vi "FTW-CodeGen-UpdateCodegenCache.vi"(5 "FTW XNode State":T1 {"TotalCodeGens" format="CodeGens:   %04d"; "TotalAdaptToInputs" format="AdaptTerms: %04d"; "FinishedCodegen" format="%_3psec"; "ElapsedTilCodegen" format="%_3psec"; "AdaptToInputsBegin" format="%.3fmsec\n%<%D:%H:%M:%S%3u>t"}, 7 "CodeGen Begin Timer":dbl format="%.3fmsec\n%<%D:%H:%M:%S%3u>t", 11 "error in":errorcluster) -> (6 "FTW XNode State out":T1 {"TotalCodeGens" format="CodeGens:   %04d"; "TotalAdaptToInputs" format="AdaptTerms: %04d"; "FinishedCodegen" format="%_3psec"; "ElapsedTilCodegen" format="%_3psec"; "AdaptToInputsBegin" format="%.3fmsec\n%<%D:%H:%M:%S%3u>t"})   [LabVIEW 2015]
uses:
  FTW-CodeGen-XNodeCommonState.ctl
  FTW-CodeGen-XNodeAdaptiveTerminal.ctl
  FTW-CodeGen-XNodeAdaptiveTerminal-Controller.ctl
  src/reflection/FTW-Reflection-Types.ctl
  FTW-CodeGen-XNodeAdaptiveTerminal-ControllerBehavior.ctl
  src/error/FTW-ERR-NoErrorConstant.vi
  lib/FTW-KernelFilepath.vi
panel:
  # "Inputs"
  # "Outputs"
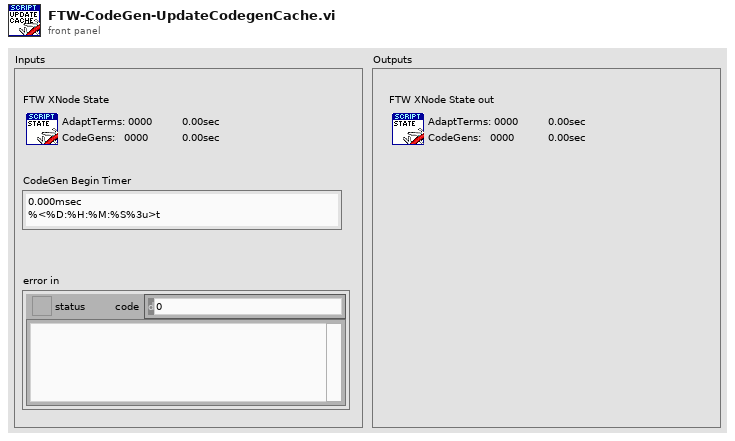
[diagram p1: front panel]
types:
  T1 = typedef "FTW-CodeGen-XNodeCommonState.ctl" = cluster{"Terms":cluster{"Name":string, "Id":string, "Type":variant, "Bounds":cluster{"Left":i32, "Top":i32, "Right":i32, "Bottom":i32}, "Input?":bool, "Required?":bool, "Recommended?":bool, "Adaptive?":bool, "Hidden?":bool, "Direction":enum32{"Auto", "Up", "Down", "Left", "Right", "Center"}, "Break Wire?":bool, "English Name":string}[], "AdaptiveTerms":T2[], "AdaptiveTerminalsOK":bool, "ForceCodeRegeneration?":bool, "LastGeneration":timestamp, "CodeGenError":errorcluster, "AdaptToInputsBegin":dbl, "ElapsedTilCodegen":dbl, "FinishedCodegen":dbl, "TotalAdaptToInputs":i32, "TotalCodeGens":i32}
  T2 = typedef "FTW-CodeGen-XNodeAdaptiveTerminal.ctl" = cluster{"Config":T3, "ID":string, "ParentIndex":i32, "Wired?":bool, "WiredTypeAllowed?":bool, "LastValidWireName":string, "LastValidWireType":T4, "Followers":i32[]}
  T3 = typedef "FTW-CodeGen-XNodeAdaptiveTerminal-Controller.ctl" = cluster{"AllowedTypes":T4[], "UnconstrainedTypeBehavior":T5, "DefaultType":variant}
  T4 = typedef "FTW-Reflection-Types.ctl" = enum16{"Unknown", "Void", "Array", "Cluster", "LVObject", "Boolean", "I8", "I16", "I32", "I64", "U8", "U16", "U32", "U64", "SGL", "DBL", "EXT", "CSG", "CDB", "CXT", "FXP", "EnumU8", "EnumU16", "EnumU32", "EnumU64", "SGLwithUnit", "DBLwithUnit", "EXTwithUnit", "CSGwithUnit", "CDBwithUnit", "CXTwithUnit", "String", "Path", "Picture", "Tag", "LVVariant", "Timestamp", "WaveformI8", "WaveformI16", "WaveformI32", "WaveformI64", "WaveformU8", "WaveformU16", "WaveformU32", "WaveformU64", "WaveformSGL", "WaveformDBL", "WaveformEXT", "WaveformCSG", "WaveformCDB", "WaveformCXT", "WaveformDigital", "WaveformUnknownType", "DigitalData", "DynamicData", "ExternalData", "FileByteStream", "TDMStream", "dotNET", "ActiveX", "VIServerReference", "VIReference", "ApplicationInstance", "Menu", "ConnectionDataSocket", "ConnectionVISA", "ConnectionBluetooth", "ConnectionIrDA", "ConnectionTCP", "ConnectionUDP", "ConnectionHTTPClient", "ConnectionFTP", "Occurrence", "Notifier", "Queue", "Rendezvous", "Semaphore", "RTFIFO", "EventPublisher", "EventRegistration", "EventCallback", "DataValueReference", "GenericClass", "GenericClassTag", "GenericClassDeepCopy", "GenericClassFlattened", "GenericClassTagFlattened", "GenericReferenceType", "WindowsRegistry", "OverloadedDatalogRef", "ReferenceUnknownType", "ByteArray", "ConPaneInterface", "FTWObject"}
  T5 = typedef "FTW-CodeGen-XNodeAdaptiveTerminal-ControllerBehavior.ctl" = enum16{"UseDefaultType", "StickyToLastValidType"}
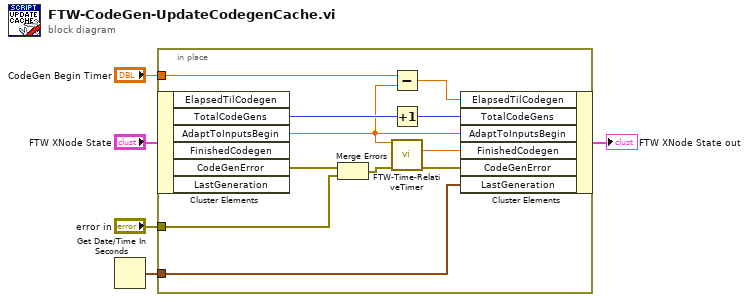
[diagram p0: block diagram]
diagram:
  n1 = Get Date/Time In Seconds() -> (seconds since 1Jan1904=w4:timestamp)
  n2 = in-place {
    in-place-border: w4 -> [w12]
    in-place-border: "error in" -> [w15]
    in-place-border: "CodeGen Begin Timer" -> [w7]
    n3 = in-place-cluster #1("FTW XNode State") -> ("TotalCodeGens"=w10:i32, "AdaptToInputsBegin"=w8:dbl, "CodeGenError"=w16:errorcluster)  [unwired: 3 out]
    n4 = Merge Errors(w16, w15) -> (w14:errorcluster)
    n5 = Subtract(x=w7, y=w8) -> (x-y=w6:dbl)
    n6 = Increment(x=w10) -> (x+1=w9:i32)
    n7 = call "FTW-Time-RelativeTimer.vi"("Previous Timer Value"=w8, "error in"=w14) -> ("Elapsed Time"=w11:dbl, "error out"=w13:errorcluster)  [unwired: 11 in, 1 out]
    n8 = in-place-cluster #1("ElapsedTilCodegen"=w6, "TotalCodeGens"=w9, "AdaptToInputsBegin"=w8, "FinishedCodegen"=w11, "CodeGenError"=w13, "LastGeneration"=w12) -> (→"FTW XNode State out":T1)
  }
